vi "GT Axis Off.vi"(8 "error in (no error)":errorcluster caption="错误输入（无错误）", 10 "axis":i16, 11 "cardNum":i16) -> (0 "error out":errorcluster caption="错误输出", 3 "cardNum":i16)   [LabVIEW 2020, in "gts.lvlib"]
doc: "GT_API GT_AxisOff(short cardNum,short axis);"
uses:
  gts.lvlib
  dll/32bit/multi_card/gts.dll
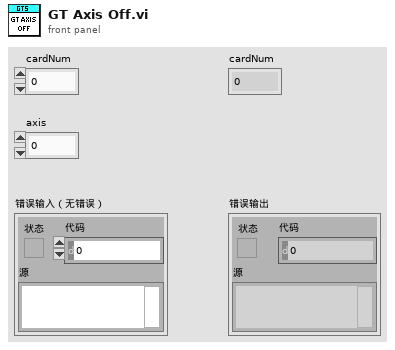
[diagram p1: front panel]
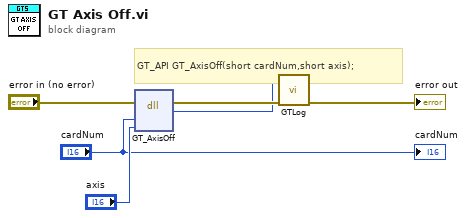
[diagram p0: block diagram]
diagram:
  # "GT_API GT_AxisOff(short cardNum,short axis);"
  n1 = dll-call lib="D:/Git/GoogolCard/dll/32bit/multi_card/gts.dll" fn="GT_AxisOff"(error in="error in (no error)", "cardNum"="cardNum", "axis"="axis") -> (error out=w4:errorcluster, w2:i16)  [unwired: 4 in, 1 out]
  n2 = call "GTLog.vi"("error in (no error)"=w4, "Numeric"=w2) -> ("error out"=→"error out":errorcluster)  [unwired: 9 in]
  "cardNum" <- "cardNum"
